vi "Case Next Frame.vi"(0 "Diagram in":refnum<vi>, 11 "error in (no error)":errorcluster) -> (4 "Selected Diagram":refnum<vi>, 6 "Selector":refnum<vi>, 8 "Inputs":refnum<vi>[](array[refnum]), 15 "error out":errorcluster)   [LabVIEW 2015, in "Scripting.lvlib"]
doc: "Navigates to the next frame of the Case Structure that owns <B>Diagram in</B>, supplying the frame's diagram at <B>Diagram out</B>. The input inside terminals and selector input terminal corresponding the diagram are output."
uses:
  Scripting.lvlib
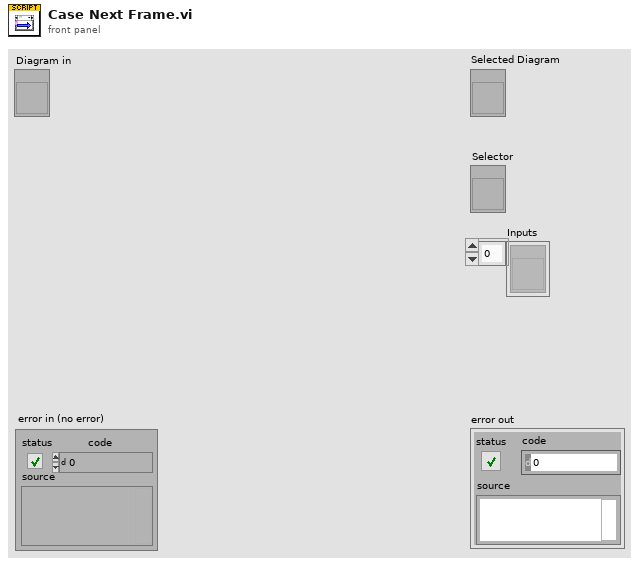
[diagram p1: front panel]
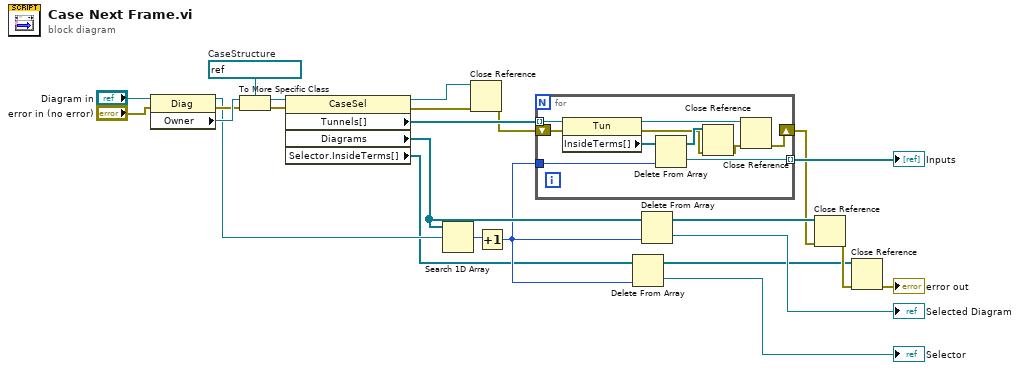
[diagram p0: block diagram]
diagram:
  w23 = refnum<vi> refnum  # CaseStructure
  n1 = property class="Diag"(reference="Diagram in", error in="error in (no error)") -> (reference out=w16:refnum<vi>, error out=w18:errorcluster, "Owner"=w19:refnum<vi>)
  n2 = To More Specific Class(target class=w23, reference=w19, error in=w18) -> (specific class reference=w11:refnum<vi>, error out=w10:errorcluster)
  n3 = property class="CaseSel"(reference=w11, error in=w10) -> (reference out=w8:refnum<vi>, error out=w7:errorcluster, "Tunnels[]"=w12:refnum<vi>[], "Diagrams"=w15:refnum<vi>[], "Selector.InsideTerms[]"=w9:refnum<vi>[])
  n4 = Search 1D Array(1D array=w15, element=w16) -> (index of element=w14:i32)  [unwired: 1 in]
  n5 = Close Reference(reference=w8, error in (no error)=w7) -> (error out=w6:errorcluster)
  n6 = Increment(x=w14) -> (x+1=w13:i32)
  n7 = for {
    tunnel: w12 -> [w34] mode=indexing
    tunnel: w13 -> [w31]
    shift-right: [w25] -> w4
    shift-left: w6 -> [w33]
    tunnel: [w30] -> w22 mode=indexing
    n8 = property class="Tun"(reference=w34, error in=w33) -> (reference out=w29:refnum<vi>, error out=w26:errorcluster, "InsideTerms[]"=w32:refnum<vi>[])
    n9 = Delete From Array(array=w32, index=w31) -> (deleted portion=w30:refnum<vi>, array with subset deleted=w27:refnum<vi>[])  [unwired: 1 in]
    n10 = Close Reference(reference=w27, error in (no error)=w26) -> (error out=w28:errorcluster)
    n11 = Close Reference(reference=w29, error in (no error)=w28) -> (error out=w25:errorcluster)
  }
  "Inputs" <- w22
  n12 = Delete From Array(array=w9, index=w13) -> (deleted portion=→"Selector":refnum<vi>, array with subset deleted=w2:refnum<vi>[])  [unwired: 1 in]
  n13 = Delete From Array(array=w15, index=w13) -> (deleted portion=→"Selected Diagram":refnum<vi>, array with subset deleted=w5:refnum<vi>[])  [unwired: 1 in]
  n14 = Close Reference(reference=w5, error in (no error)=w4) -> (error out=w3:errorcluster)
  n15 = Close Reference(reference=w2, error in (no error)=w3) -> (error out=→"error out":errorcluster)
